vi "Dequeue Element.vi"(6 "timeout in ms (-1)":i32=-1, 8 "error in":errorcluster, 11 "QueueMessageTransport in":refnum<class "QueueMessageTransport.lvclass">) -> (0 "error out":errorcluster, 2 "Q Element":refnum<class "IMessagePayload.lvclass">, 3 "QueueMessageTransport out":refnum<class "QueueMessageTransport.lvclass">)   [LabVIEW 2016, in "QueueMessageTransport.lvclass"]
uses:
  QueueMessageTransport.lvclass
  IMessagePayload/IMessagePayload.lvclass
  QueueMessageTransport.lvclass/QueueMessageTransport.ctl
panel:
  # "INPUTS"
  # "OUTPUTS"
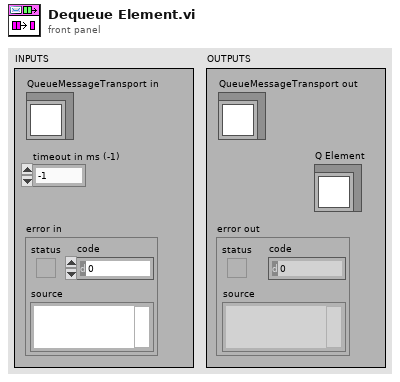
[diagram p1: front panel]
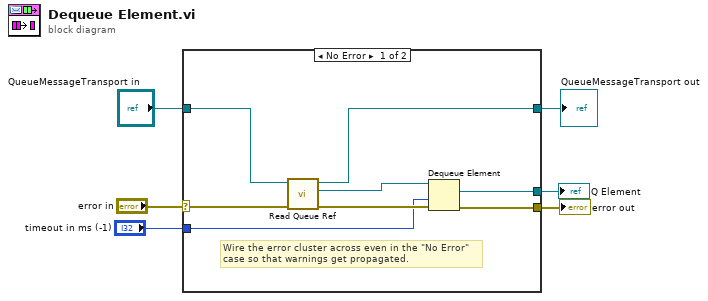
[diagram p0: block diagram]
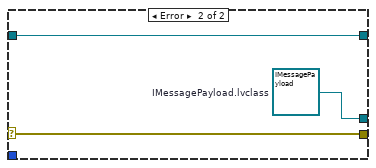
[diagram p2: hidden frame]
diagram:
  n1 = case shown="No Error" "error in" {
    selector: "error in" -> [w14 w17]
    tunnel: [w8 w17] -> w5
    tunnel: [w12 w16] -> w3
    tunnel: "QueueMessageTransport in" -> [w13 w16]
    tunnel: "timeout in ms (-1)" -> [w9 _]
    tunnel: [w7 w15] -> w1
    frame No Error {
      # "Wire the error cluster across even in the \"No Error\"\ncase so that warnings get propagated."
      n2 = call "Read Queue Ref.vi"("error in"=w14, "QueueMessageTransport in"=w13) -> ("error out"=w11:errorcluster, "Queue Ref"=w10:refnum<queue>, "QueueMessageTransport out"=w12:refnum<class "QueueMessageTransport.lvclass">)  [unwired: 7 in]
      n3 = Dequeue Element(queue=w10, timeout in ms (-1)=w9, error in (no error)=w11) -> (element=w7:refnum<class "IMessagePayload.lvclass">, error out=w8:errorcluster)  [unwired: 2 out]
    }
    frame Error {
      w15 = refnum<class "IMessagePayload.lvclass"> refnum  # IMessagePayload.lvclass
    }
  }
  "error out" <- w5
  "QueueMessageTransport out" <- w3
  "Q Element" <- w1
